vi "运维调试_CODCr.vi"() -> ()   [LabVIEW 2016, in "CODCr库.lvlib"]
uses:
  <vilib>/Utility/miscctls.llb/LVPointTypeDef.ctl
  <vilib>/ptbypt/NI_PtbyPt.lvlib
  <vilib>/Utility/config.llb/NI_LVConfig.lvlib
panel:
  in  "仪器参数":bool
  in  "MB通信方式选择":enum16{"串口", "TCP"}(ring)
  in  "释放串口":bool
  in  "打开串口":bool
  in  "加标回收测试":bool
  in  "平行样测试":bool
  in  "定时启动":bool
  out "COM口":string
  in  "空白测试":bool
  in  "隐藏按钮":bool
  in  "写入消解温度时长":bool
  in  "保存KB值":bool
  in  "标样核查":bool
  out "启动时间":timestamp format="%<%Y/%m/%d %H:%M:%S>T"
  out "主循环次数":i32
  out "status":bool
  out "启动测量模式":T1(ring)
  out "曲线斜率B":sgl format="%#_10g"
  out "曲线斜率K":sgl format="%#_10g"
  out "量程上限":sgl
  out "量程下限":sgl
  out "消解时长":u16
  out "消解温度":u16
  out "测量精度":u16
  out "测量结果":sgl
  out "标样参考值":sgl
  out "量程":u16
  out "工作状态":T1(ring)
  out "仪器时间":timestamp format="%<%X\n%x>T"
  out "关键参数区":T2
  out "状态告警区":T3
  out "测量数据区":T4 {"单位" items=["ug/L", "mg/L", "ppm", "mg/m3", "cm", "ppb", "ug/m3", "%", "nmol/mol", "umol/mol", "MPN/L", "MPN/100ml", "ng/m3", "NTU", "无量纲", "ms/cm", "us/cm", "℃", "mV", "万个/L"]}
  out "系统时间":timestamp format="%<%Y/%m/%d %H:%M:%S>T"
  in  "停止":bool
  in  "校时":bool
  in  "标样校准":bool
  in  "空白校准":bool
  in  "零点核查":bool
  in  "跨度核查":bool
  in  "水样测试":bool
  in  "返回":bool
  in  "设置":bool
  # "mg/L"
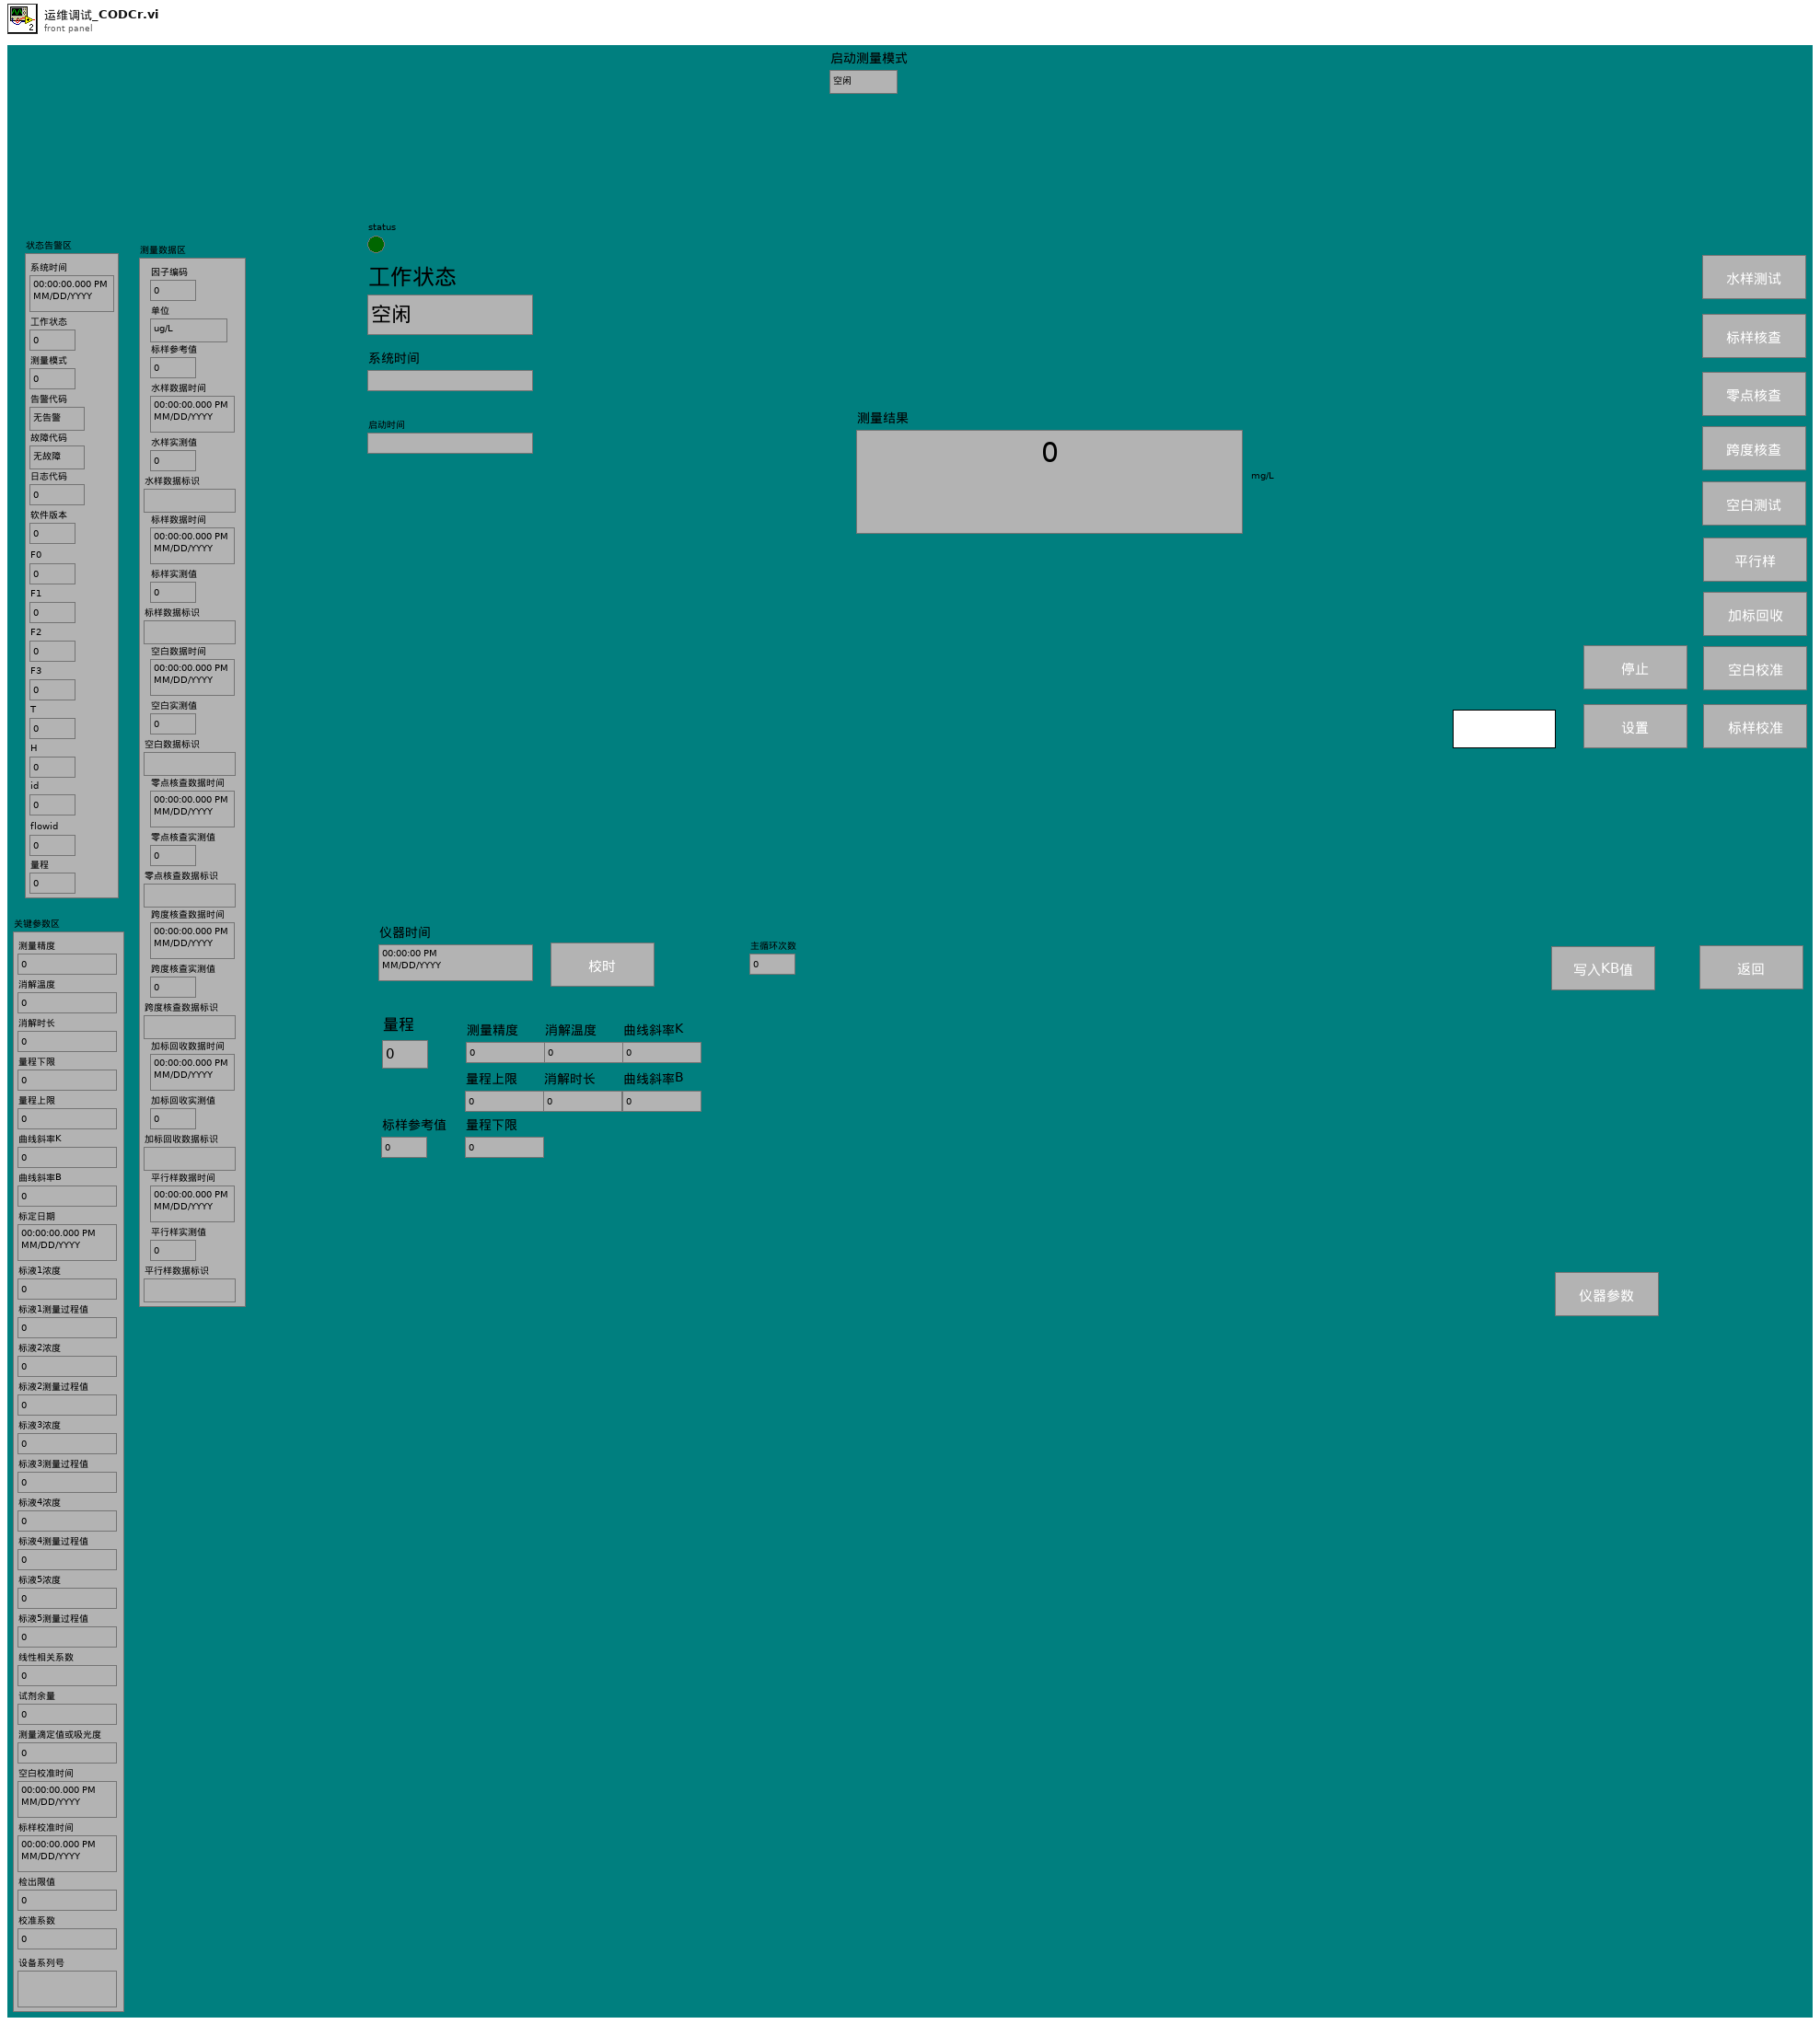
[diagram p1: front panel]
types:
  T1 = enum16{"空闲", "水样测试", "标样核查", "零点核查", "跨度核查", "空白测试", "平行样测试", "加标回收", "空白校准", "标样校准", "初始化（清洗）"}
  T2 = cluster{"测量精度":u16, "消解温度":u16, "消解时长":u16, "量程下限":sgl, "量程上限":sgl, "曲线斜率K":sgl, "曲线斜率B":sgl, "标定日期":timestamp, "标液1浓度":sgl, "标液1测量过程值":sgl, "标液2浓度":sgl, "标液2测量过程值":sgl, "标液3浓度":sgl, "标液3测量过程值":sgl, "标液4浓度":sgl, "标液4测量过程值":sgl, "标液5浓度":sgl, "标液5测量过程值":sgl, "线性相关系数":sgl, "试剂余量":u32, "测量滴定值或吸光度":sgl, "空白校准时间":timestamp, "标样校准时间":timestamp, "检出限值":sgl, "校准系数":sgl, "设备系列号":string}
  T3 = cluster{"系统时间":timestamp, "工作状态":u16, "测量模式":u16, "告警代码":enum16{"无告警", "缺试剂告警", "缺水样告警", "缺蒸馏水告警", "缺标液告警", "仪表漏液告警", "标定异常告警", "超量程告警", "加热异常", "低试剂预警", "超上限告警", "超下限告警", "仪表内部其他异常", "滴定异常告警", "电极异常告警", "量程切换告警", "参数设置告警", "PH电极电位异常", "电导率电极异常", "浊度光度异常", "溶解氧电极异常", "溶解氧光强异常", "温度异常告警", "PH异常告警", "溶解氧异常告警", "电导率异常告警", "浊度异常告警", "叶绿素异常告警", "藻密度异常告警", "蓝绿藻异常告警", "ORP异常告警", "氨氮异常告警", "清洁刷异常告警", "SD卡异常告警", "蓝牙异常告警", "Wifi异常告警", "流程异常告警"}, "故障代码":enum16{"无故障", "电机故障", "温度故障", "通讯故障", "滴定故障"}, "日志代码":u16, "软件版本":u16, "F0":sgl, "F1":sgl, "F2":sgl, "F3":sgl, "T":sgl, "H":sgl, "id":u16, "flowid":u16, "量程":u16}
  T4 = cluster{"因子编码":u32, "单位":u16, "标样参考值":sgl, "水样数据时间":timestamp, "水样实测值":sgl, "水样数据标识":string, "标样数据时间":timestamp, "标样实测值":sgl, "标样数据标识":string, "空白数据时间":timestamp, "空白实测值":sgl, "空白数据标识":string, "零点核查数据时间":timestamp, "零点核查实测值":sgl, "零点核查数据标识":string, "跨度核查数据时间":timestamp, "跨度核查实测值":sgl, "跨度核查数据标识":string, "加标回收数据时间":timestamp, "加标回收实测值":sgl, "加标回收数据标识":string, "平行样数据时间":timestamp, "平行样实测值":sgl, "平行样数据标识":string}
  T5 = cluster{"命令":string, "测量模式":enum16{"水样测量", "标样核查", "零点核查", "跨度核查", "空白测试", "加标回收", "平行样", "校零", "校标"}, "CODCr量程切换":enum32{"H", "L", "AUTO"}}
  T6 = cluster{"测量模式":enum16{"水样测量", "标样核查", "零点核查", "跨度核查", "空白测试", "加标回收", "平行样", "校零", "校标"}}
  T7 = cluster{"仪器测试类型":enum16{"水样测试", "标样核查", "空白测试", "跨度核查"}, "周期设置类型":enum16{"定点启动", "间隔启动"}, "定时功能启用":bool, "定时间隔":dbl, "24H周期设置":bool[]}
  T8 = typedef "LVDateTimeRec.ctl" = cluster{"秒数的小数部分":dbl, "秒":i32, "分":i32, "时":i32, "日":i32, "月":i32, "年":i32, "天数（周）":i32, "天数（年）":i32, "DST":i32}
  T9 = typedef "LVPointTypeDef.ctl" = cluster{"Horizontal":i16, "Vertical":i16}
  T10 = typedef "NI_LVConfig.lvlib/Config Data RefNum.ctl" = refnum<k1>
  T11 = cluster{"运行模式":enum16{"维护模式", "常规模式", "应急模式", "质控模式"}}
  T12 = cluster{"时间标识":timestamp, "监测值":sgl, "单位":u16, "数据标识":string, "因子编码":u32, "标样参考值":sgl, "F0":sgl, "F1":sgl, "F2":sgl, "F3":sgl, "温度":sgl, "湿度":sgl, "量程标识":string}
  T13 = cluster{"时间标识":timestamp, "设备":string, "日志信息":string}
  T14 = cluster{"时间标识":timestamp, "参数":string, "日志信息":string, "流程参数":string}
  T15 = enum16{"无告警", "缺试剂告警", "缺水样告警", "缺蒸馏水告警", "缺标液告警", "仪表漏液告警", "标定异常告警", "超量程告警", "加热异常", "低试剂预警", "超上限告警", "超下限告警", "仪表内部其他异常", "滴定异常告警", "电极异常告警", "量程切换告警", "参数设置告警", "PH电极电位异常", "电导率电极异常", "浊度光度异常", "溶解氧电极异常", "溶解氧光强异常", "温度异常告警", "PH异常告警", "溶解氧异常告警", "电导率异常告警", "浊度异常告警", "叶绿素异常告警", "藻密度异常告警", "蓝绿藻异常告警", "ORP异常告警", "氨氮异常告警", "清洁刷异常告警", "SD卡异常告警", "蓝牙异常告警", "Wifi异常告警", "流程异常告警"}
  T16 = cluster{"时间标识":timestamp, "设备":string, "日志信息":string, "流程参数":string}
  T17 = enum16{"水样测量", "标样核查", "零点核查", "跨度核查", "空白测试", "加标回收", "平行样", "校零", "校标"}
  T18 = cluster{"测量量程":dbl, "测量精度":dbl, "测量间隔":dbl, "消解温度":dbl, "消解时长":dbl, "空白校准时间":timestamp, "曲线截距":dbl, "曲线斜率":dbl, "测量检出限":dbl, "测量信号值":dbl, "线性相关系数":dbl, "二次多项式系数":dbl, "标样校准时间":timestamp, "单位":u16}
  T19 = cluster{"确定":bool, "测量量程":dbl, "测量精度":dbl, "测量间隔":dbl, "消解温度":dbl, "消解时长":dbl, "空白校准时间":timestamp, "曲线截距":dbl, "曲线斜率":dbl, "测量检出限":dbl, "测量信号值":dbl, "线性相关系数":dbl, "二次多项式系数":dbl, "标样校准时间":timestamp, "单位":u16}
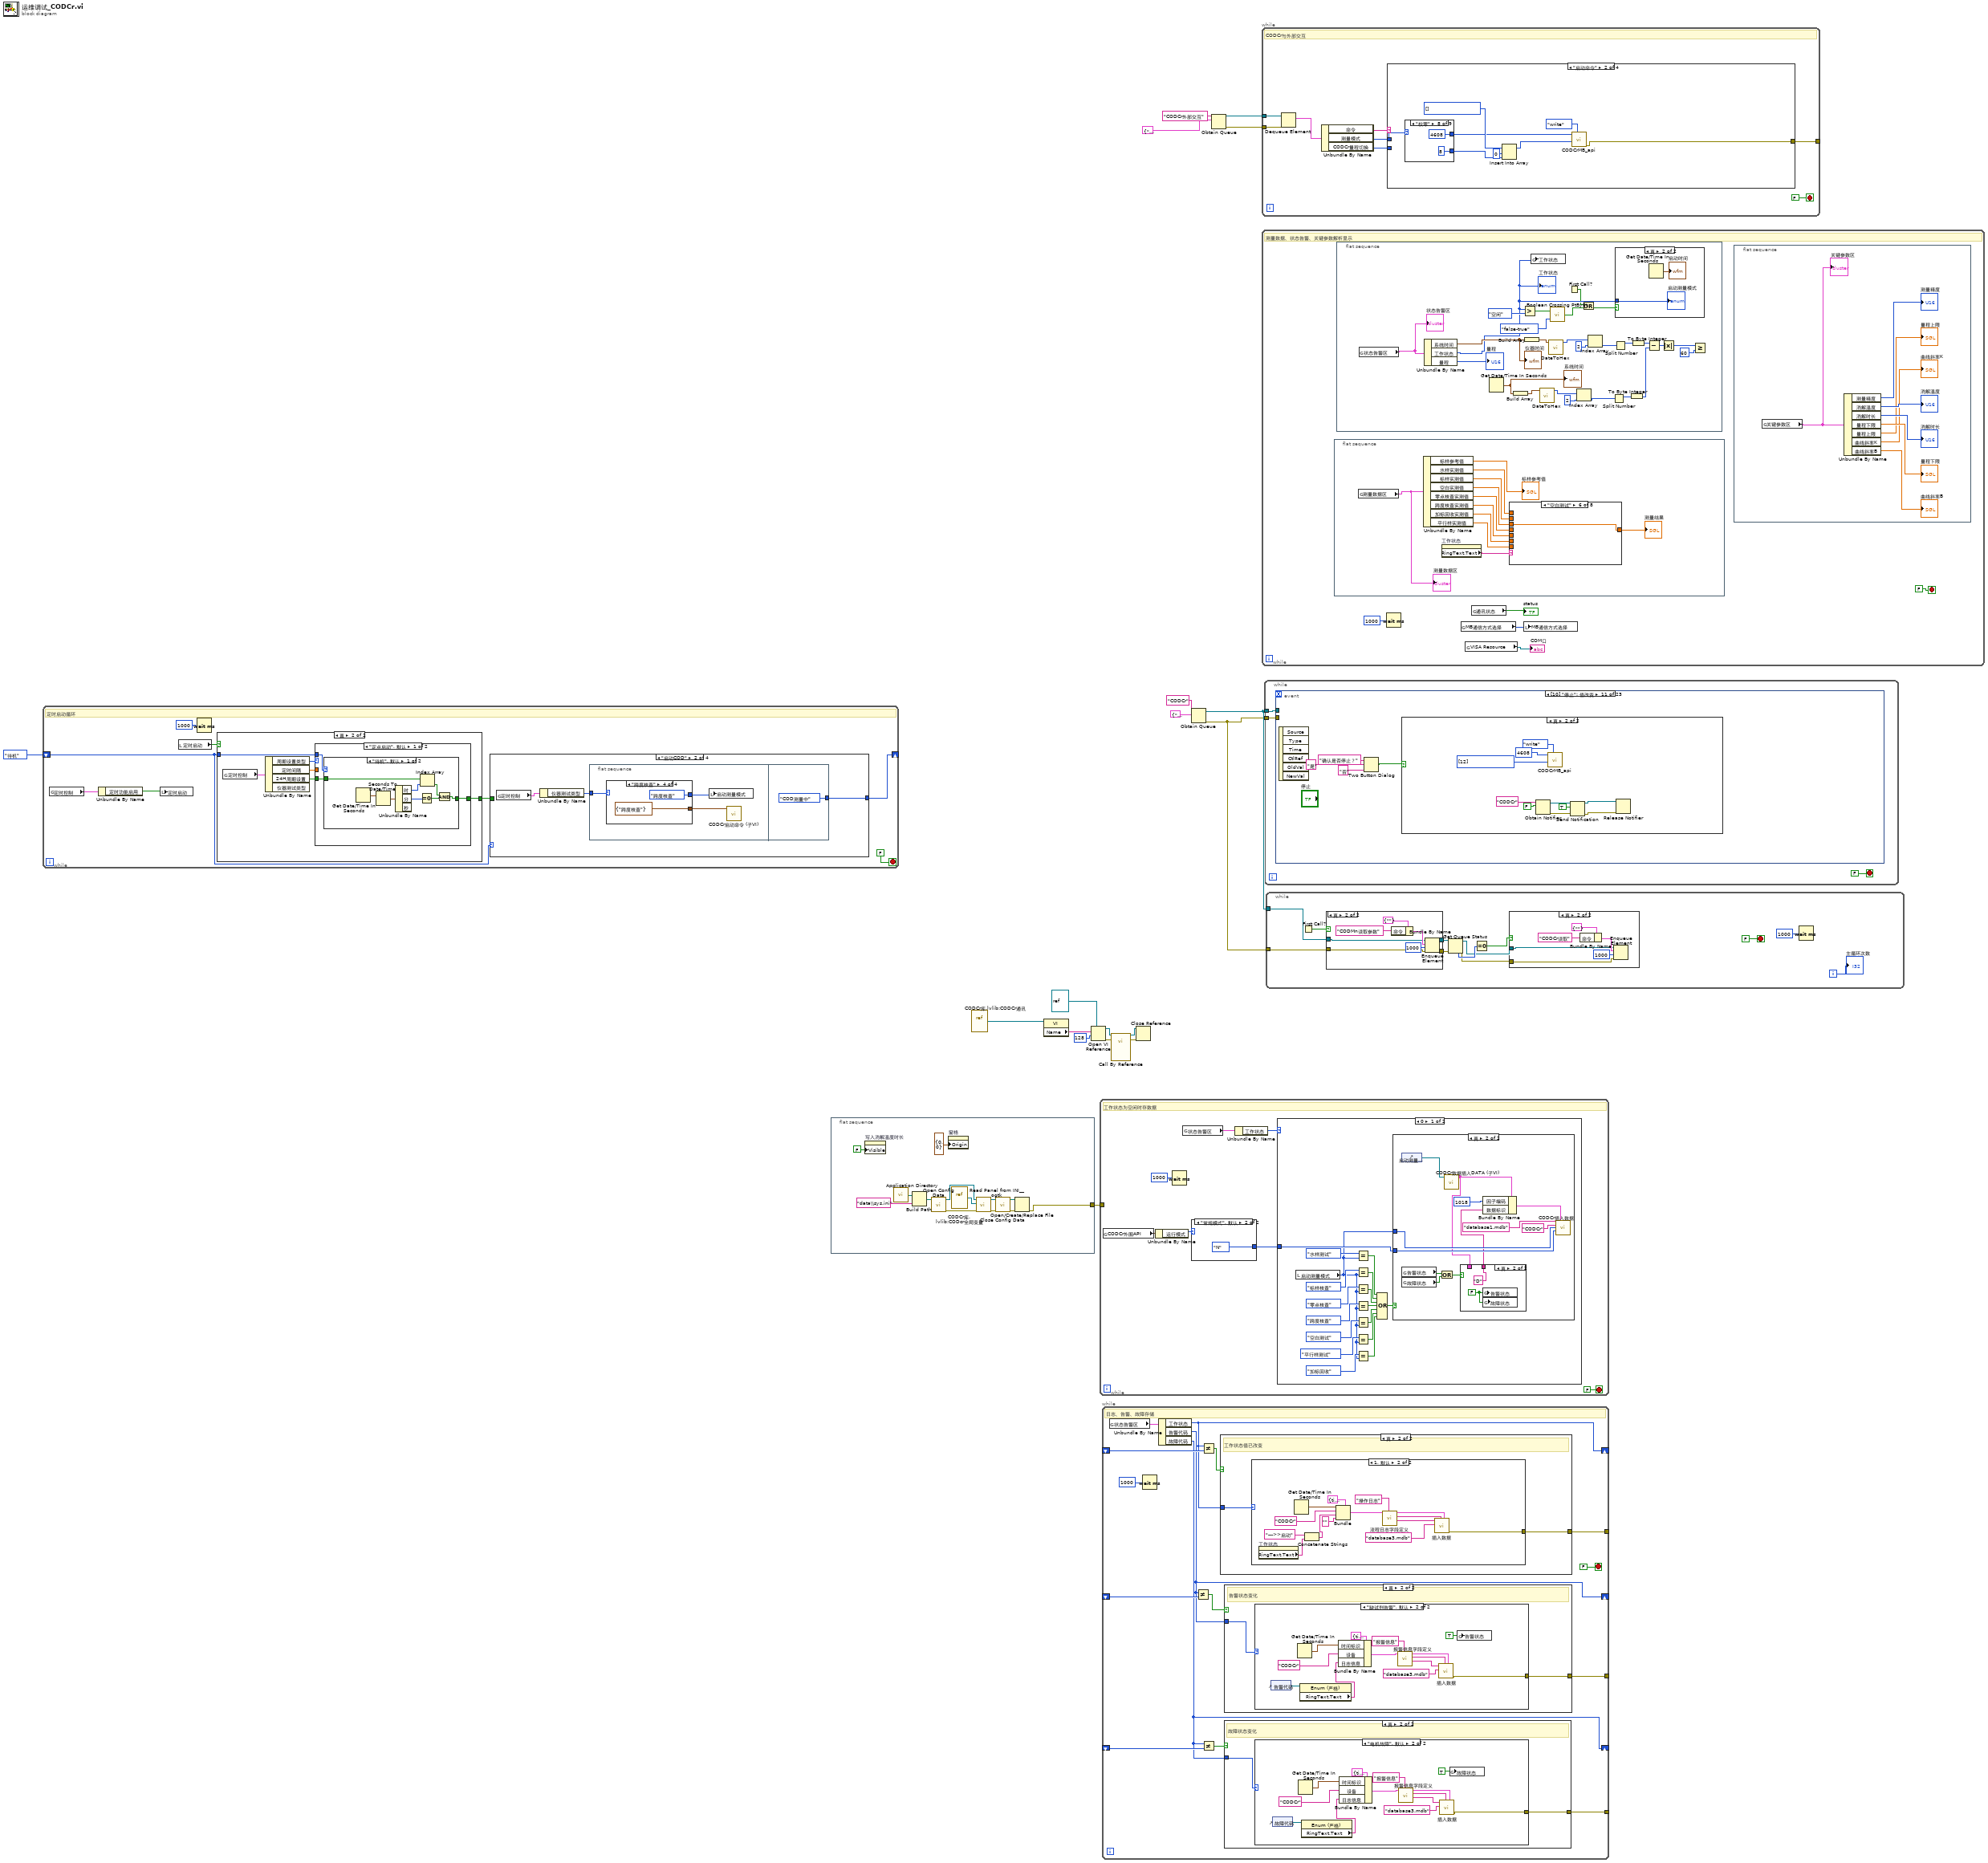
[diagram p0: block diagram]
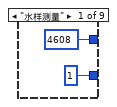
[diagram p5: hidden frame]
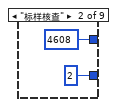
[diagram p6: hidden frame]
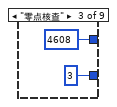
[diagram p7: hidden frame]
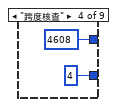
[diagram p8: hidden frame]
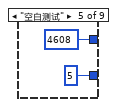
[diagram p9: hidden frame]
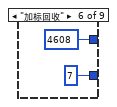
[diagram p10: hidden frame]
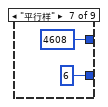
[diagram p11: hidden frame]
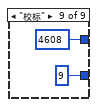
[diagram p12: hidden frame]
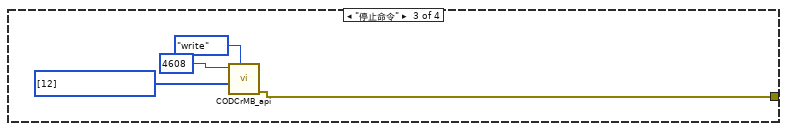
[diagram p13: hidden frame]
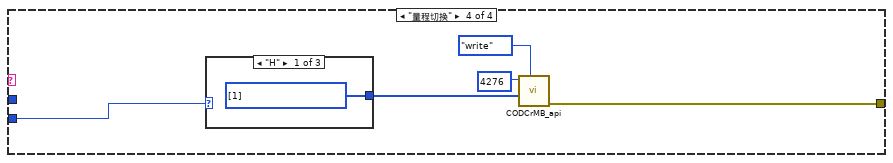
[diagram p14: hidden frame]
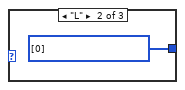
[diagram p15: hidden frame]
diagram:
  n1 = while {
    shift-right: [w24] -> _
    shift-left: enum16{"待机", "启动COD", "COD测量中", "延时"}."待机" -> [w23]
    stop <- FALSE stop-if-true
    # "定时启动循环"
    n2 = global read "CODcr全局变量.vi" "定时控制"() -> (w20:T7)
    n3 = Unbundle By Name(w20) -> ("定时功能启用"=w19:bool)
    n4 = local write "定时启动"(w19) -> ()
    n5 = local read "定时启动"() -> (w21:bool)
    n6 = Wait (ms)(milliseconds to wait=u32 1000 ("等待时间（毫秒）")) -> ()  [unwired: 1 out]
    n7 = case shown="真" w21 {
      tunnel: w23 -> [_ w59]
      tunnel: [_ w58] -> w22
      frame False {
      }
      frame True {
        n8 = global read "CODcr全局变量.vi" "定时控制"() -> (w57:T7)
        n9 = Unbundle By Name(w57) -> ("周期设置类型"=w60:enum16{"定点启动", "间隔启动"}, "定时间隔"=w61:dbl, "24H周期设置"=w62:bool[])  [unwired: 1 out]
        n10 = case shown="\"定点启动\", 默认" w60 {
          tunnel: w61 -> [_ w77]
          tunnel: w62 -> [w65 _]
          tunnel: w59 -> [w63 w80]
          tunnel: [w64 w75] -> w58
          frame "定点启动", Default {
            n11 = case shown="\"待机\", 默认" w63 {
              tunnel: w65 -> [w71 _]
              tunnel: [w66 _] -> w64
              frame "待机", Default {
                n12 = Get Date/Time In Seconds() -> (seconds since 1Jan1904=w73:timestamp)
                n13 = Seconds To Date/Time(time stamp (now)=w73) -> (date time rec=w72:T8)  [unwired: 1 in]
                n14 = Unbundle By Name(w72) -> ("时"=w70:i32, "分"=w69:i32)  [unwired: 1 out]
                n15 = Equal To 0?(x=w69) -> (x = 0?=w67:bool)
                n16 = Index Array(array=w71, index=w70) -> (element=w68:bool)
                n17 = Compound Arithmetic op=AND ("复合运算")(w68, w67) -> (w66:bool)
              }
              frame "启动COD" {
              }
            }
          }
          frame "间隔启动" {
            n18 = Multiply(x=w77, y=60.0) -> (x*y=w74:dbl)
            n19 = feedback #1(w74) -> (w79:dbl)
            n20 = case shown="\"待机\"" w80 {
              tunnel: w79 -> [_ w82]
              tunnel: [_ w81] -> w78
              frame Default {
              }
              frame "待机" {
                n21 = Increment(x=w82) -> (x+1=w81:dbl)
              }
            }
            n22 = feedback-in #1(w78) -> ()
            n23 = Greater Or Equal?(x=w78, y=w74) -> (x >= y?=w75:bool)
          }
        }
      }
    }
    n24 = case shown="\"启动COD\"" w23 {
      tunnel: [w27 w33 w47 enum16{"待机", "启动COD", "COD测量中", "延时"}."待机"] -> w24
      tunnel: w22 -> [w30 _ _ _]
      frame "待机", Default {
        n25 = Select(t=enum16{"待机", "启动COD", "COD测量中", "延时"}."启动COD", s=w30, f=enum16{"待机", "启动COD", "COD测量中", "延时"}."待机") -> (s? t:f=w27:enum16{"待机", "启动COD", "COD测量中", "延时"})
      }
      frame "启动COD" {
        n26 = global read "CODcr全局变量.vi" "定时控制"() -> (w31:T7)
        n27 = Unbundle By Name(w31) -> ("仪器测试类型"=w32:enum16{"水样测试", "标样核查", "空白测试", "跨度核查"})
        n28 = flat-sequence {
          tunnel: w32 -> [w36]
          tunnel: [enum16{"待机", "启动COD", "COD测量中", "延时"}."COD测量中"] -> w33
          frame #0 {
            n29 = case shown="\"跨度核查\"" w36 {
              tunnel: [T6 {"测量模式"=enum."水样测量"} ("启动测量模式") T6 {"测量模式"=enum."标样核查"} ("启动测量模式") T6 {"测量模式"=enum."空白测试"} ("启动测量模式") T6 {"测量模式"=enum."跨度核查"} ("启动测量模式")] -> w35
              tunnel: [T1."水样测试" ("启动测量模式") T1."标样核查" ("启动测量模式") T1."空白测试" ("启动测量模式") T1."跨度核查" ("启动测量模式")] -> w34
              frame "水样测试", Default {
              }
              frame "标样核查" {
              }
              frame "空白测试" {
              }
              frame "跨度核查" {
              }
            }
            n30 = local write "启动测量模式"(w34) -> ()
            n31 = call "CODCr启动命令 (子VI).vi"("启动测量模式"=w35) -> ()  [unwired: 11 in]
          }
          frame #1 {
          }
        }
      }
      frame "COD测量中" {
        n32 = flat-sequence {
          tunnel: [w51] -> w46
          tunnel: [w55] -> w47
          tunnel: w46 -> [w55]
          frame #0 {
            n33 = local read "状态告警区"() -> (w50:T3)
            n34 = Unbundle By Name(w50) -> ("工作状态"=w49:u16)
            n35 = Equal To 0?(x=w49) -> (x = 0?=w48:bool)
            n36 = Select(t=enum16{"待机", "启动COD", "COD测量中", "延时"}."延时", s=w48, f=enum16{"待机", "启动COD", "COD测量中", "延时"}."COD测量中") -> (s? t:f=w51:enum16{"待机", "启动COD", "COD测量中", "延时"})
          }
          frame #1 {
            n37 = Wait (ms)(milliseconds to wait=u32 5000 ("等待时间（毫秒）")) -> ()  [unwired: 1 out]
          }
        }
      }
      frame "延时" {
      }
    }
  }
  n38 = flat-sequence {
    tunnel: [w83] -> w17
    frame #0 {
      n39 = property on="写入消解温度时长" class="Bool"("Visible"=FALSE ("可见")) -> ()  [unwired: 2 in, 2 out]
      n40 = call <vilib>:"Application Directory.vi"() -> ("Application Directory"=w93:path)
      n41 = Build Path(base path=w93, name or relative path="data\\sys.ini" ("名称或相对路径")) -> (appended path=w91:path)
      n42 = call <vilib>:"Open Config Data.vi"("configuration file path"=w91) -> ("error out"=w87:errorcluster, "refnum"=w90:T10)  [unwired: 8 in, 1 out]
      n43 = property on="窗格" class="Pane"("Origin"=T9 {"Horizontal"=0, "Vertical"=0} ("原点")) -> ()  [unwired: 2 in, 2 out]
      n44 = vi-ref "CODCr库.lvlib:CODcr全局变量.vi"() -> (w89:refnum<vi>)
      n45 = call <userlib>:"Read Panel from INI__ogtk.vi"("error in (no error)"=w87, "VI ref"=w89, "refnum"=w90) -> ("error out"=w86:errorcluster, "refnum out"=w88:T10)  [unwired: 7 in]
      n46 = call <vilib>:"Close Config Data.vi"("error in (no error)"=w86, "refnum"=w88) -> ("error out"=w85:errorcluster, "file path"=w84:path)  [unwired: 8 in]
      n47 = Open/Create/Replace File(file path (use dialog)=w84, error in=w85) -> (error out=w83:errorcluster)  [unwired: 4 in, 2 out]
    }
  }
  n48 = vi-ref "CODCr库.lvlib:CODCr通讯.vi"() -> (w9:refnum<vi>)
  n49 = property class="VI"(reference=w9) -> ("Name"=w10:string)  [unwired: 1 in, 2 out]
  n50 = Open VI Reference(type specifier VI Refnum (for type only)=refnum<vi> refnum, vi path=w10, options=128 ("选项")) -> (vi reference=w12:refnum<vi>, error out=w14:errorcluster)  [unwired: 3 in]
  n51 = while "While循环" {
    tunnel: w17 -> [_]
    stop <- FALSE stop-if-true
    # "工作状态为空闲时存数据"
    n52 = global read "CODCr外部API.vi" "CODCr外围API"() -> (w98:T11)
    n53 = Unbundle By Name(w98) -> ("运行模式"=w97:enum16{"维护模式", "常规模式", "应急模式", "质控模式"})
    n54 = Wait (ms)(milliseconds to wait=u32 1000 ("等待时间（毫秒）")) -> ()  [unwired: 1 out]
    n55 = global read "CODcr全局变量.vi" "状态告警区"() -> (w96:T3)
    n56 = case shown="\"常规模式\", 默认" w97 {
      tunnel: [enum16{"N", "M"}."M" ("数据类型") enum16{"N", "M"}."N" ("数据类型")] -> w99
      frame "维护模式" {
      }
      frame "常规模式", Default {
      }
    }
    n57 = Unbundle By Name(w96) -> ("工作状态"=w100:u16)
    n58 = case shown="0" w100 {
      tunnel: w99 -> [w121 _]
      frame 0 {
        n59 = local read "启动测量模式"() -> (w113:T1)
        n60 = Equal?(x=T1."水样测试" ("启动测量模式"), y=w113) -> (x = y?=w112:bool)
        n61 = Equal?(x=T1."标样核查" ("启动测量模式"), y=w113) -> (x = y?=w111:bool)
        n62 = Equal?(x=T1."零点核查" ("启动测量模式"), y=w113) -> (x = y?=w110:bool)
        n63 = Equal?(x=T1."跨度核查" ("启动测量模式"), y=w113) -> (x = y?=w109:bool)
        n64 = Equal?(x=T1."空白测试" ("启动测量模式"), y=w113) -> (x = y?=w108:bool)
        n65 = Equal?(x=T1."平行样测试" ("启动测量模式"), y=w113) -> (x = y?=w107:bool)
        n66 = Equal?(x=T1."加标回收" ("启动测量模式"), y=w113) -> (x = y?=w106:bool)
        n67 = Compound Arithmetic op=OR(w112, w111, w110, w109, w108, w107, w106) -> (w105:bool)
        n68 = case shown="真" w105 {
          tunnel: w113 -> [_ w129]
          tunnel: w121 -> [_ w128]
          frame False {
          }
          frame True {
            n69 = control-ref of="启动测量模式"() -> (w133:refnum<vi>)
            n70 = global read "CODcr全局变量.vi" "告警状态"() -> (w126:bool)
            n71 = global read "CODcr全局变量.vi" "故障状态"() -> (w125:bool)
            n72 = Or(x=w126, y=w125) -> (x .or. y?=w124:bool)
            n73 = call "CODCr数据插入DATA (子VI).vi"("Enum输入"=w133) -> ("data"=w123:T12)  [unwired: 10 in]
            n74 = case shown="真" w124 {
              tunnel: w123 -> [w135 _]
              tunnel: [w134 "D" ("table")] -> w122
              frame False {
                n75 = Unbundle By Name(w135) -> ("数据标识"=w134:string)
              }
              frame True {
                w136 = FALSE ("告警状态")
                n76 = global write "CODcr全局变量.vi" "告警状态"(w136) -> ()
                n77 = global write "CODcr全局变量.vi" "故障状态"(w136) -> ()
              }
            }
            n78 = Bundle By Name(cluster=w123, "因子编码"=u32 1018, "数据标识"=w122) -> (w132:T12)
            n79 = call "CODCr插入数据.vi"("database"="database1.mdb", "data"=w132, "table"="CODCr", "测量模式"=w129, "数据类型"=w128) -> ()  [unwired: 10 in, 1 out]
          }
        }
      }
      frame 1, Default {
      }
    }
  }
  n80 = while {
    shift-right: [w148] -> _
    shift-left: _ -> [w150]
    tunnel: [w147] -> _
    shift-right: [w143] -> _
    shift-left: _ -> [w144]
    shift-right: [w139] -> _
    shift-left: _ -> [w141]
    tunnel: [w140] -> _
    tunnel: [w138] -> _
    stop <- FALSE stop-if-true
    # "日志、告警、故障存储"
    n81 = global read "CODcr全局变量.vi" "状态告警区"() -> (w146:T3)
    n82 = Wait (ms)(milliseconds to wait=u32 1000 ("等待时间（毫秒）")) -> ()  [unwired: 1 out]
    n83 = Unbundle By Name(w146) -> ("工作状态"=w148:u16, "告警代码"=w143:T15, "故障代码"=w139:enum16{"无故障", "电机故障", "温度故障", "通讯故障", "滴定故障"})
    n84 = Not Equal?(x=w143, y=w144) -> (x != y?=w145:bool)
    n85 = Not Equal?(x=w148, y=w150) -> (x != y?=w149:bool)
    n86 = Not Equal?(x=w139, y=w141) -> (x != y?=w142:bool)
    n87 = case shown="真" w149 {
      tunnel: w148 -> [_ w184]
      tunnel: [_ w183] -> w147
      frame False {
      }
      frame True {
        # "工作状态值已改变"
        n88 = case shown="1, 默认" w184 {
          tunnel: [w185 w200] -> w183
          frame 0 {
            n89 = Get Date/Time In Seconds() -> (seconds since 1Jan1904=w192:timestamp)
            n90 = Bundle(cluster=T14 {"时间标识"=timestamp(0 s since 1904-01-01), "参数"="", "日志信息"="", "流程参数"=""} ("data in"), "时间标识"=w192, "参数"="CODCr" ("table输入"), "日志信息"="--->>结束", "流程参数"="" ("table输入")) -> (w186:T14)
            n91 = call "流程日志字段定义.vi"("table输入"="操作日志", "data in"=w186) -> ("table输出"=w190:string, "columns"=w188:string[], "data out"=w187:T16)  [unwired: 7 in]
            n92 = call "插入数据.vi"("data"=w187, "columns"=w188, "database"="database3.mdb", "table"=w190) -> ("error out"=w185:errorcluster)  [unwired: 7 in]
          }
          frame 1, Default {
            n93 = property on="工作状态" class="Enum (严格)"() -> ("RingText.Text"=w197:string)  [unwired: 2 in, 2 out]
            n94 = Get Date/Time In Seconds() -> (seconds since 1Jan1904=w207:timestamp)
            n95 = Concatenate Strings("--->>启动" ("日志信息"), w197) -> (w198:string)
            n96 = Bundle(cluster=T14 {"时间标识"=timestamp(0 s since 1904-01-01), "参数"="", "日志信息"="", "流程参数"=""} ("data in"), "时间标识"=w207, "参数"="CODCr" ("table输入"), "日志信息"=w198, "流程参数"="" ("table输入")) -> (w206:T14)
            n97 = call "流程日志字段定义.vi"("table输入"="操作日志", "data in"=w206) -> ("table输出"=w204:string, "columns"=w202:string[], "data out"=w201:T16)  [unwired: 7 in]
            n98 = call "插入数据.vi"("data"=w201, "columns"=w202, "database"="database3.mdb", "table"=w204) -> ("error out"=w200:errorcluster)  [unwired: 7 in]
          }
        }
      }
    }
    n99 = case shown="真" w142 {
      tunnel: w139 -> [_ w154]
      tunnel: [_ w153] -> w138
      frame False {
      }
      frame True {
        # "故障状态变化"
        n100 = case shown="\"电机故障\", 默认" w154 {
          tunnel: [_ w156] -> w153
          frame "无故障" {
            # "无告警"
          }
          frame "电机故障", Default {
            n101 = control-ref of="故障代码"() -> (w166:refnum<vi>)
            n102 = Get Date/Time In Seconds() -> (seconds since 1Jan1904=w164:timestamp)
            n103 = property class="Enum (严格)"(reference=w166) -> ("RingText.Text"=w167:string)  [unwired: 1 in, 2 out]
            n104 = Bundle By Name(cluster=T13 {"时间标识"=timestamp(0 s since 1904-01-01), "设备"="", "日志信息"=""} ("data in"), "时间标识"=w164, "设备"="CODCr" ("table输入"), "日志信息"=w167) -> (w163:T13)
            n105 = call "报警信息字段定义.vi"("table输入"="报警信息", "data in"=w163) -> ("table输出"=w158:string, "columns"=w157:string[], "data out"=w160:T13)  [unwired: 7 in]
            n106 = call "插入数据.vi"("data"=w160, "columns"=w157, "database"="database3.mdb", "table"=w158) -> ("error out"=w156:errorcluster)  [unwired: 7 in]
            n107 = global write "CODcr全局变量.vi" "故障状态"(TRUE ("告警状态")) -> ()
          }
        }
      }
    }
    n108 = case shown="真" w145 {
      tunnel: w143 -> [_ w169]
      tunnel: [_ w168] -> w140
      frame False {
      }
      frame True {
        # "告警状态变化"
        n109 = case shown="\"缺试剂告警\", 默认" w169 {
          tunnel: [_ w175] -> w168
          frame "无告警" {
            # "无告警"
          }
          frame "缺试剂告警", Default {
            n110 = control-ref of="告警代码"() -> (w172:refnum<vi>)
            n111 = Get Date/Time In Seconds() -> (seconds since 1Jan1904=w174:timestamp)
            n112 = property class="Enum (严格)"(reference=w172) -> ("RingText.Text"=w171:string)  [unwired: 1 in, 2 out]
            n113 = Bundle By Name(cluster=T13 {"时间标识"=timestamp(0 s since 1904-01-01), "设备"="", "日志信息"=""} ("data in"), "时间标识"=w174, "设备"="CODCr" ("table输入"), "日志信息"=w171) -> (w176:T13)
            n114 = call "报警信息字段定义.vi"("table输入"="报警信息", "data in"=w176) -> ("table输出"=w181:string, "columns"=w182:string[], "data out"=w179:T13)  [unwired: 7 in]
            n115 = call "插入数据.vi"("data"=w179, "columns"=w182, "database"="database3.mdb", "table"=w181) -> ("error out"=w175:errorcluster)  [unwired: 7 in]
            n116 = global write "CODcr全局变量.vi" "告警状态"(TRUE ("告警状态")) -> ()
          }
        }
      }
    }
  }
  n117 = call-by-ref "?"(reference=w12, error in=w14) -> (reference out=w16:refnum<vi>, error out=w15:errorcluster)  [unwired: 12 in]
  n118 = Close Reference(reference=w16, error in (no error)=w15) -> ()  [unwired: 1 out]
  n119 = Obtain Queue(name (unnamed)="CODCr" ("名称（未命名）"), element data type=cluster{"命令":string} {"命令"="启用模块"} ("元素")) -> (queue out=w2:refnum<queue>, error out=w1:errorcluster)  [unwired: 3 in, 1 out]
  n120 = Obtain Queue(name (unnamed)="CODCr外部交互" ("名称（未命名）"), element data type=T5 {"命令"="启动命令", "测量模式"=enum."水样测量", "CODCr量程切换"=enum."AUTO"} ("元素")) -> (queue out=w4:refnum<queue>, error out=w3:errorcluster)  [unwired: 3 in, 1 out]
  n121 = while {
    tunnel: w4 -> [w216]
    tunnel: w3 -> [w215]
    tunnel: [w211] -> _
    stop <- FALSE stop-if-true
    # "CODCr与外部交互"
    n122 = Dequeue Element(queue=w216, error in (no error)=w215) -> (element=w217:T5)  [unwired: 1 in, 3 out]
    n123 = Unbundle By Name(w217) -> ("命令"=w214:string, "测量模式"=w213:T17, "CODCr量程切换"=w212:enum32{"H", "L", "AUTO"})
    n124 = case shown="\"启动命令\"" w214 {
      tunnel: w213 -> [_ w220 _ _]
      tunnel: w212 -> [_ _ _ w250]
      tunnel: [_ w219 w245 w249] -> w211
      frame "假", Default {
      }
      frame "启动命令" {
        n125 = case shown="\"校零\"" w220 {
          tunnel: [u16 4608 ("address") u16 4608 ("address") u16 4608 ("address") u16 4608 ("address") u16 4608 ("address") u16 4608 ("address") u16 4608 ("address") u16 4608 ("address") u16 4608 ("address")] -> w222
          tunnel: [u16 1 ("address") u16 2 ("address") u16 3 ("address") u16 4 ("address") u16 5 ("address") u16 7 ("address") u16 6 ("address") u16 8 ("address") u16 9 ("address")] -> w226
          frame "水样测量" {
          }
          frame "标样核查" {
          }
          frame "零点核查" {
          }
          frame "跨度核查" {
          }
          frame "空白测试" {
          }
          frame "加标回收" {
          }
          frame "平行样" {
          }
          frame "校零" {
          }
          frame "校标" {
          }
        }
        n126 = Insert Into Array(array=u16[] [] ("values"), index=0 ("索引"), new element=w226) -> (w221:u16[])
        n127 = call "CODCrMB_api.vi"("STEP"=enum16{"open", "read", "write", "close"}."write", "values"=w221, "starting address"=w222) -> ("error out"=w219:errorcluster)  [unwired: 6 in, 2 out]
      }
      frame "停止命令" {
        n128 = call "CODCrMB_api.vi"("STEP"=enum16{"open", "read", "write", "close"}."write", "values"=u16[] [12], "starting address"=u16 4608) -> ("error out"=w245:errorcluster)  [unwired: 6 in, 2 out]
      }
      frame "量程切换" {
        n129 = case shown="\"H\"" w250 {
          tunnel: [u16[] [1] ("values") u16[] [0] ("values") _] -> w253
          frame "H" {
          }
          frame "L" {
          }
          frame "AUTO", Default {
          }
        }
        n130 = call "CODCrMB_api.vi"("STEP"=enum16{"open", "read", "write", "close"}."write", "values"=w253, "starting address"=u16 4276) -> ("error out"=w249:errorcluster)  [unwired: 6 in, 2 out]
      }
    }
  }
  n131 = while {
    stop <- FALSE stop-if-true
    # "测量数据、状态告警、关键参数解析显示"
    n132 = flat-sequence {
      frame #0 {
        n133 = global read "CODcr全局变量.vi" "测量数据区"() -> (w297:T4)
        "测量数据区" <- w297
        n134 = Unbundle By Name(w297) -> ("标样参考值"=→"标样参考值":sgl, "水样实测值"=w305:sgl, "标样实测值"=w303:sgl, "空白实测值"=w300:sgl, "零点核查实测值"=w302:sgl, "跨度核查实测值"=w301:sgl, "加标回收实测值"=w298:sgl, "平行样实测值"=w299:sgl)
        n135 = property on="工作状态" class="Enum (严格)"() -> ("RingText.Text"=w306:string)  [unwired: 2 in, 2 out]
        n136 = case shown="\"空白测试\"" w306 {
          tunnel: w305 -> [_ w309 _ _ _ _ _ _]
          tunnel: [w308 w309 w310 w311 w312 w313 w314 w315] -> w304
          tunnel: w303 -> [_ _ w310 _ _ _ _ _]
          tunnel: w302 -> [_ _ _ w311 _ _ _ _]
          tunnel: w301 -> [_ _ _ _ w312 _ _ _]
          tunnel: w300 -> [_ _ _ _ _ w313 _ _]
          tunnel: w299 -> [_ _ _ _ _ _ w314 _]
          tunnel: w298 -> [_ _ _ _ _ _ _ w315]
          frame "空闲", Default {
            n137 = local read "测量结果"() -> (w308:sgl)
          }
          frame "水样测试" {
          }
          frame "标样核查" {
          }
          frame "零点核查" {
          }
          frame "跨度核查" {
          }
          frame "空白测试" {
          }
          frame "平行样测试" {
          }
          frame "加标回收" {
          }
        }
        "测量结果" <- w304
      }
    }
    n138 = flat-sequence {
      frame #0 {
        n139 = global read "CODcr全局变量.vi" "状态告警区"() -> (w269:T3)
        "状态告警区" <- w269
        n140 = Unbundle By Name(w269) -> ("系统时间"=w281:timestamp, "工作状态"=w272:u16, "量程"=→"量程":u16)
        "仪器时间" <- w281
        "工作状态" <- w272
        n141 = Get Date/Time In Seconds() -> (seconds since 1Jan1904=w282:timestamp)
        "系统时间" <- w282
        n142 = Build Array(w282) -> (w276:timestamp[])
        n143 = Greater?(x=w272, y=T1."空闲") -> (0:w280:bool)
        n144 = Build Array(w281) -> (w275:timestamp[])
        n145 = global write "CODcr全局变量.vi" "工作状态"(w272) -> ()
        n146 = call "DateToHex.vi"("DATE"=w276) -> ("数组"=w273:u16[])  [unwired: 10 in]
        n147 = call "DateToHex.vi"("DATE"=w275) -> ("数组"=w274:u16[])  [unwired: 10 in]
        n148 = call <vilib>:"Boolean Crossing PtByPt.vi"("direction"=enum16{"either", "false-true", "true-false"}."false-true", "input"=w280) -> ("crossing"=w279:bool)  [unwired: 1 in]
        n149 = First Call?() -> (First Call?: T/F=w270:bool)
        n150 = Index Array(array=w273, index=2 ("索引")) -> (element=w284:u16)
        n151 = Or(x=w270, y=w279) -> (x .or. y?=w271:bool)
        n152 = Index Array(array=w274, index=2 ("索引")) -> (element=w285:u16)
        n153 = Split Number(x=w284) -> (hi(x)=w287:u8)  [unwired: 1 out]
        n154 = Split Number(x=w285) -> (hi(x)=w290:u8)  [unwired: 1 out]
        n155 = case shown="真" w271 {
          tunnel: w272 -> [_ w295]
          frame False {
          }
          frame True {
            n156 = Get Date/Time In Seconds() -> (seconds since 1Jan1904=→"启动时间":timestamp)
            "启动测量模式" <- w295
          }
        }
        n157 = To Byte Integer(number=w287) -> (8bit integer=w288:i8)
        n158 = To Byte Integer(number=w290) -> (8bit integer=w291:i8)
        n159 = Subtract(x=w291, y=w288) -> (x-y=w289:i8)
        n160 = Absolute Value(x=w289) -> (abs(x)=w292:i8)
        n161 = Greater Or Equal?(x=w292, y=i8 60) -> ()  [unwired: 1 out]
      }
    }
    n162 = Wait (ms)(milliseconds to wait=u32 1000 ("等待时间（毫秒）")) -> ()  [unwired: 1 out]
    n163 = global read "CODcr全局变量.vi" "MB通信方式选择"() -> (w257:enum16{"串口", "TCP"})
    n164 = global read "CODcr全局变量.vi" "VISA Resource"() -> (→"COM口":refnum<visa-resource-name>)
    n165 = global read "CODcr全局变量.vi" "通讯状态"() -> (→"status":bool)
    n166 = local write "MB通信方式选择"(w257) -> ()
    n167 = flat-sequence {
      frame #0 {
        n168 = global read "CODcr全局变量.vi" "关键参数区"() -> (w261:T2)
        "关键参数区" <- w261
        n169 = Unbundle By Name(w261) -> ("测量精度"=→"测量精度":u16, "消解温度"=→"消解温度":u16, "消解时长"=→"消解时长":u16, "量程下限"=→"量程下限":sgl, "量程上限"=→"量程上限":sgl, "曲线斜率K"=→"曲线斜率K":sgl, "曲线斜率B"=→"曲线斜率B":sgl)
      }
    }
  }
  n170 = while {
    tunnel: w2 -> [w317]
    tunnel: w1 -> [w316]
    stop <- FALSE stop-if-true
    n171 = event shown="[10] \"停止\": 值改变" {
      selector: _ -> [_ _ _ _ _ _ _ _ _ _ _ _ _ _ _ _ _ _ _ _ _ _ _]
      dyn-events: _ -> [_ _ _ _ _ _ _ _ _ _ _ _ _ _ _ _ _ _ _ _ _ _ _]
      timeout: _ -> [_ _ _ _ _ _ _ _ _ _ _ _ _ _ _ _ _ _ _ _ _ _ _]
      tunnel: w317 -> [_ _ _ _ _ _ _ _ _ _ _ _ _ _ w428 w445 _ _ _ w483 _ _ _]
      tunnel: w316 -> [_ _ _ _ _ _ _ _ _ _ _ _ _ _ w427 w444 _ _ _ w482 _ _ _]
      event Timeout {
        n172 = event-data() -> ()  [unwired: 1 in, 2 out]
      }
      event "水样测试": Value Change {
        n173 = event-data() -> ()  [unwired: 1 in, 6 out]
        n174 = local write "启动测量模式"(T1."水样测试" ("启动测量模式")) -> ()
        n175 = call "CODCrMB_api.vi"("STEP"=enum16{"open", "read", "write", "close"}."write", "values"=u16[] [1], "starting address"=u16 4608) -> ()  [unwired: 6 in, 3 out]
      }
      event "标样核查": Value Change {
        n176 = event-data() -> ()  [unwired: 1 in, 6 out]
        n177 = local write "启动测量模式"(T1."标样核查" ("启动测量模式")) -> ()
        n178 = call "CODCrMB_api.vi"("STEP"=enum16{"open", "read", "write", "close"}."write", "values"=u16[] [2], "starting address"=u16 4608) -> ()  [unwired: 6 in, 3 out]
      }
      event "零点核查": Value Change {
        n179 = event-data() -> ()  [unwired: 1 in, 6 out]
        n180 = local write "启动测量模式"(T1."零点核查" ("启动测量模式")) -> ()
        n181 = call "CODCrMB_api.vi"("STEP"=enum16{"open", "read", "write", "close"}."write", "values"=u16[] [3], "starting address"=u16 4608) -> ()  [unwired: 6 in, 3 out]
      }
      event "跨度核查": Value Change {
        n182 = event-data() -> ()  [unwired: 1 in, 6 out]
        n183 = local write "启动测量模式"(T1."跨度核查" ("启动测量模式")) -> ()
        n184 = call "CODCrMB_api.vi"("STEP"=enum16{"open", "read", "write", "close"}."write", "values"=u16[] [4], "starting address"=u16 4608) -> ()  [unwired: 6 in, 3 out]
      }
      event "空白测试": Value Change {
        n185 = event-data() -> ()  [unwired: 1 in, 6 out]
        n186 = local write "启动测量模式"(T1."空白测试" ("启动测量模式")) -> ()
        n187 = call "CODCrMB_api.vi"("STEP"=enum16{"open", "read", "write", "close"}."write", "values"=u16[] [5], "starting address"=u16 4608) -> ()  [unwired: 6 in, 3 out]
      }
      event "平行样测试": Value Change {
        n188 = event-data() -> ()  [unwired: 1 in, 6 out]
        n189 = local write "启动测量模式"(T1."平行样测试" ("启动测量模式")) -> ()
        n190 = call "CODCrMB_api.vi"("STEP"=enum16{"open", "read", "write", "close"}."write", "values"=u16[] [6], "starting address"=u16 4608) -> ()  [unwired: 6 in, 3 out]
      }
      event "加标回收测试": Value Change {
        n191 = event-data() -> ()  [unwired: 1 in, 6 out]
        n192 = local write "启动测量模式"(T1."加标回收" ("启动测量模式")) -> ()
        n193 = call "CODCrMB_api.vi"("STEP"=enum16{"open", "read", "write", "close"}."write", "values"=u16[] [7], "starting address"=u16 4608) -> ()  [unwired: 6 in, 3 out]
      }
      event "空白校准": Value Change {
        n194 = event-data() -> ()  [unwired: 1 in, 6 out]
        n195 = local write "启动测量模式"(T1."空白校准" ("启动测量模式")) -> ()
        n196 = call "CODCrMB_api.vi"("STEP"=enum16{"open", "read", "write", "close"}."write", "values"=u16[] [8], "starting address"=u16 4608) -> ()  [unwired: 6 in, 3 out]
      }
      event "标样校准": Value Change {
        n197 = event-data() -> ()  [unwired: 1 in, 6 out]
        n198 = local write "启动测量模式"(T1."标样校准" ("启动测量模式")) -> ()
        n199 = call "CODCrMB_api.vi"("STEP"=enum16{"open", "read", "write", "close"}."write", "values"=u16[] [9], "starting address"=u16 4608) -> ()  [unwired: 6 in, 3 out]
      }
      event "停止": Value Change {
        n200 = event-data() -> ()  [unwired: 1 in, 6 out]
        n201 = Two Button Dialog(message="确认是否停止？" ("消息"), 1:"否" ("F按钮名称（“取消”）"), 2:"是" ("T按钮名称（“确定”）")) -> (T button?=w355:bool)
        n202 = case shown="真" w355 {
          frame False {
          }
          frame True {
            n203 = Obtain Notifier(name (unnamed)="CODCr" ("名称（未命名）"), notification data type=FALSE) -> (notifier out=w363:refnum<notifier>, error out=w361:errorcluster)  [unwired: 2 in, 1 out]
            n204 = call "CODCrMB_api.vi"("STEP"=enum16{"open", "read", "write", "close"}."write", "values"=u16[] [12], "starting address"=u16 4608) -> ()  [unwired: 6 in, 3 out]
            n205 = Send Notification(notification=TRUE ("通知"), notifier=w363, error in (no error)=w361) -> (notifier out=w360:refnum<notifier>, error out=w359:errorcluster)
            n206 = Release Notifier(notifier=w360, error in (no error)=w359) -> ()  [unwired: 1 in, 3 out]
          }
        }
      }
      event "保存KB值": Value Change {
        n207 = event-data() -> ()  [unwired: 1 in, 6 out]
        n208 = local read "曲线斜率B"() -> (w373:sgl)
        n209 = local read "曲线斜率K"() -> (w374:sgl)
        n210 = Build Array(w374, w373) -> (w372:sgl[])
        n211 = call "FloatToHex.vi"("浮点数"=w372) -> ("DCBA整形输出"=w369:u16[])  [unwired: 10 in]
        n212 = call "CODCrMB_api.vi"("STEP"=enum16{"open", "read", "write", "close"}."write", "values"=w369, "starting address"=u16 4263) -> ()  [unwired: 6 in, 3 out]
      }
      event "定时启动": Value Change {
        n213 = event-data() -> ()  [unwired: 1 in, 6 out]
        n214 = flat-sequence {
          frame #0 {
            n215 = global read "CODcr全局变量.vi" "定时控制"() -> (w376:T7)
            n216 = call "周期设置.vi"("定时控制参数输入"=w376) -> ("定时控制参数输出"=w375:T7)  [unwired: 10 in]
            n217 = global write "CODcr全局变量.vi" "定时控制"(w375) -> ()
          }
          frame #1 {
            n218 = call <vilib>:"Application Directory.vi"() -> ("Application Directory"=w390:path)
            n219 = Build Path(base path=w390, name or relative path="data\\sys.ini" ("名称或相对路径")) -> (appended path=w388:path)
            n220 = call <vilib>:"Open Config Data.vi"("configuration file path"=w388) -> ("error out"=w384:errorcluster, "refnum"=w387:T10)  [unwired: 8 in, 1 out]
            n221 = vi-ref "CODCr库.lvlib:CODcr全局变量.vi"() -> (w386:refnum<vi>)
            n222 = call <userlib>:"Write Panel to INI__ogtk.vi"("error in (no error)"=w384, "VI ref"=w386, "refnum"=w387) -> ("error out"=w383:errorcluster, "refnum out"=w385:T10)  [unwired: 7 in]
            n223 = call <vilib>:"Close Config Data.vi"("error in (no error)"=w383, "refnum"=w385) -> ("error out"=w378:errorcluster, "file path"=w377:path)  [unwired: 8 in]
            n224 = Open/Create/Replace File(file path (use dialog)=w377, error in=w378) -> (refnum out=w381:refnum<file>, error out=w382:errorcluster)  [unwired: 4 in, 1 out]
            n225 = Flush File(refnum=w381, error in=w382) -> (refnum out=w380:refnum<file>, error out=w379:errorcluster)
            n226 = Close File(refnum=w380, error in=w379) -> ()  [unwired: 2 out]
          }
        }
      }
      event "仪器参数": Value Change {
        n227 = event-data() -> ()  [unwired: 1 in, 6 out]
        n228 = global read "CODcr全局变量.vi" "CODCr仪器参数"() -> (w392:T18)
        n229 = call "仪器参数设置.vi"("仪器参数设置"=w392) -> ("仪器参数设置输出"=w391:T19)  [unwired: 10 in]
        n230 = Unbundle By Name(w391) -> ("确定"=w393:bool)
        n231 = case shown="真" w393 {
          tunnel: w392 -> [_ w395]
          tunnel: w391 -> [_ w394]
          frame False {
          }
          frame True {
            n232 = flat-sequence {
              tunnel: w395 -> [w412]
              tunnel: w394 -> [w411]
              frame #0 {
                n233 = Unbundle By Name(w411) -> ("测量量程"=w410:dbl, "测量精度"=w409:dbl, "测量间隔"=w408:dbl, "消解温度"=w407:dbl, "消解时长"=w406:dbl, "空白校准时间"=w405:timestamp, "曲线截距"=w404:dbl, "曲线斜率"=w403:dbl, "测量检出限"=w402:dbl, "测量信号值"=w401:dbl, "线性相关系数"=w400:dbl, "二次多项式系数"=w399:dbl, "标样校准时间"=w398:timestamp, "单位"=w397:u16)
                n234 = Bundle By Name(cluster=w412, "测量量程"=w410, "测量精度"=w409, "测量间隔"=w408, "消解温度"=w407, "消解时长"=w406, "空白校准时间"=w405, "曲线截距"=w404, "曲线斜率"=w403, "测量检出限"=w402, "测量信号值"=w401, "线性相关系数"=w400, "二次多项式系数"=w399, "标样校准时间"=w398, "单位"=w397) -> (w396:T18)
                n235 = global write "CODcr全局变量.vi" "CODCr仪器参数"(w396) -> ()
              }
              frame #1 {
                n236 = call <vilib>:"Application Directory.vi"() -> ("Application Directory"=w426:path)
                n237 = Build Path(base path=w426, name or relative path="data\\sys.ini" ("名称或相对路径")) -> (appended path=w424:path)
                n238 = call <vilib>:"Open Config Data.vi"("configuration file path"=w424) -> ("error out"=w420:errorcluster, "refnum"=w423:T10)  [unwired: 8 in, 1 out]
                n239 = vi-ref "CODCr库.lvlib:CODcr全局变量.vi"() -> (w422:refnum<vi>)
                n240 = call <userlib>:"Write Panel to INI__ogtk.vi"("error in (no error)"=w420, "VI ref"=w422, "refnum"=w423) -> ("error out"=w419:errorcluster, "refnum out"=w421:T10)  [unwired: 7 in]
                n241 = call <vilib>:"Close Config Data.vi"("error in (no error)"=w419, "refnum"=w421) -> ("error out"=w414:errorcluster, "file path"=w413:path)  [unwired: 8 in]
                n242 = Open/Create/Replace File(file path (use dialog)=w413, error in=w414) -> (refnum out=w417:refnum<file>, error out=w418:errorcluster)  [unwired: 4 in, 1 out]
                n243 = Flush File(refnum=w417, error in=w418) -> (refnum out=w416:refnum<file>, error out=w415:errorcluster)
                n244 = Close File(refnum=w416, error in=w415) -> ()  [unwired: 2 out]
              }
            }
          }
        }
      }
      event "打开串口": Value Change {
        n245 = event-data() -> ()  [unwired: 1 in, 6 out]
        n246 = global read "CODcr全局变量.vi" "VISA Resource"() -> (w435:refnum<visa-resource-name>)
        n247 = global read "CODcr全局变量.vi" "PORT"() -> (w429:string)
        n248 = global read "CODcr全局变量.vi" "IP"() -> (w430:string)
        n249 = call "串口配置.vi"("PORT"=w429, "IP"=w430, "请选择串口:"=w435) -> ("PORT 2"=w431:string, "IP 2"=w432:string, "确认 2"=w434:bool, "VISA资源名称 2"=w433:refnum<visa-resource-name>)  [unwired: 5 in]
        n250 = case shown="真" w434 {
          tunnel: w433 -> [_ w438]
          tunnel: w428 -> [_ w440]
          tunnel: w427 -> [_ w439]
          tunnel: w432 -> [_ w437]
          tunnel: w431 -> [_ w436]
          frame False {
          }
          frame True {
            n251 = global write "CODcr全局变量.vi" "VISA Resource"(w438) -> ()
            n252 = global write "CODcr全局变量.vi" "PORT"(w436) -> ()
            n253 = global write "CODcr全局变量.vi" "IP"(w437) -> ()
            n254 = Bundle By Name(cluster=cluster{"命令":string} {"命令"=""} ("元素"), "命令"="启用模块" ("名称（未命名）")) -> (w441:cluster{"命令":string})
            n255 = Enqueue Element(queue=w440, element=w441, error in (no error)=w439) -> ()  [unwired: 1 in, 3 out]
          }
        }
      }
      event "释放串口": Value Change {
        n256 = event-data() -> ()  [unwired: 1 in, 6 out]
        n257 = Two Button Dialog(message="确认是否释放串口，释放串口将导致通信失败！" ("消息")) -> (T button?=w446:bool)  [unwired: 2 in]
        n258 = case shown="真" w446 {
          tunnel: w445 -> [_ w449]
          tunnel: w444 -> [_ w448]
          frame False {
          }
          frame True {
            n259 = Bundle By Name(cluster=cluster{"命令":string} {"命令"=""} ("元素"), "命令"="停用模块" ("名称（未命名）")) -> (w450:cluster{"命令":string})
            n260 = Enqueue Element(queue=w449, element=w450, error in (no error)=w448) -> ()  [unwired: 1 in, 3 out]
          }
        }
      }
      event "MB通信方式选择": Value Change {
        n261 = event-data() -> ()  [unwired: 1 in, 6 out]
        n262 = flat-sequence {
          frame #0 {
            n263 = global write "CODcr全局变量.vi" "MB通信方式选择"("MB通信方式选择") -> ()
          }
          frame #1 {
            n264 = call <vilib>:"Application Directory.vi"() -> ("Application Directory"=w467:path)
            n265 = Build Path(base path=w467, name or relative path="data\\sys.ini" ("名称或相对路径")) -> (appended path=w465:path)
            n266 = call <vilib>:"Open Config Data.vi"("configuration file path"=w465) -> ("error out"=w461:errorcluster, "refnum"=w464:T10)  [unwired: 8 in, 1 out]
            n267 = vi-ref "CODCr库.lvlib:CODcr全局变量.vi"() -> (w463:refnum<vi>)
            n268 = call <userlib>:"Write Panel to INI__ogtk.vi"("error in (no error)"=w461, "VI ref"=w463, "refnum"=w464) -> ("error out"=w460:errorcluster, "refnum out"=w462:T10)  [unwired: 7 in]
            n269 = call <vilib>:"Close Config Data.vi"("error in (no error)"=w460, "refnum"=w462) -> ("error out"=w455:errorcluster, "file path"=w454:path)  [unwired: 8 in]
            n270 = Open/Create/Replace File(file path (use dialog)=w454, error in=w455) -> (refnum out=w458:refnum<file>, error out=w459:errorcluster)  [unwired: 4 in, 1 out]
            n271 = Flush File(refnum=w458, error in=w459) -> (refnum out=w457:refnum<file>, error out=w456:errorcluster)
            n272 = Close File(refnum=w457, error in=w456) -> ()  [unwired: 2 out]
          }
        }
      }
      event "写入消解温度时长": Value Change {
        n273 = event-data() -> ()  [unwired: 1 in, 6 out]
        n274 = local read "消解时长"() -> (w472:u16)
        n275 = local read "消解温度"() -> (w473:u16)
        n276 = Build Array(w473, w472) -> (w471:u16[])
        n277 = call "WordToHex.vi"("WORD"=w471) -> ("数组"=w468:u16[])  [unwired: 10 in]
        n278 = call "CODCrMB_api.vi"("STEP"=enum16{"open", "read", "write", "close"}."write", "values"=w468, "starting address"=u16 4257) -> ()  [unwired: 6 in, 3 out]
      }
      event "校时": Value Change {
        n279 = event-data() -> ()  [unwired: 1 in, 6 out]
        n280 = Get Date/Time In Seconds() -> (seconds since 1Jan1904=w481:timestamp)
        n281 = Build Array(w481) -> (w478:timestamp[])
        n282 = call "DateToHex.vi"("DATE"=w478) -> ("数组"=w477:u16[])  [unwired: 10 in]
        n283 = Insert Into Array(array=u16[] [13] ("values"), index=1 ("索引"), new element=w477) -> (w474:u16[])
        n284 = call "CODCrMB_api.vi"("STEP"=enum16{"open", "read", "write", "close"}."write", "values"=w474, "starting address"=u16 4608) -> ()  [unwired: 6 in, 3 out]
      }
      event "设置": Value Change {
        n285 = event-data() -> ()  [unwired: 1 in, 6 out]
        n286 = property on="窗格" class="Pane"("Origin"=T9 {"Horizontal"=0, "Vertical"=728} ("原点")) -> ()  [unwired: 2 in, 2 out]
        n287 = Bundle By Name(cluster=cluster{"命令":string} {"命令"=""} ("元素"), "命令"="CODCr读取参数" ("名称（未命名）")) -> (w484:cluster{"命令":string})
        n288 = Enqueue Element(queue=w483, element=w484, error in (no error)=w482) -> ()  [unwired: 1 in, 3 out]
      }
      event "返回": Value Change {
        w488 = FALSE ("可见")
        n289 = event-data() -> ()  [unwired: 1 in, 6 out]
        n290 = property on="窗格" class="Pane"("Origin"=T9 {"Horizontal"=0, "Vertical"=0} ("原点")) -> ()  [unwired: 2 in, 2 out]
        n291 = property on="写入消解温度时长" class="Bool"("Visible"=w488) -> ()  [unwired: 2 in, 2 out]
        n292 = property on="释放串口" class="Bool"("Visible"=w488) -> ()  [unwired: 2 in, 2 out]
        n293 = property on="打开串口" class="Bool"("Visible"=w488) -> ()  [unwired: 2 in, 2 out]
        n294 = property on="MB通信方式选择" class="Enum (严格)"("Visible"=w488) -> ()  [unwired: 2 in, 2 out]
      }
      event "曲线斜率K", "曲线斜率B", "消解温度", "消解时长": Mouse Down {
        n295 = event-data() -> ("CtlRef"=w492:refnum<vi>)  [unwired: 1 in, 7 out]
        n296 = property class="DigNum"(reference=w492) -> (reference out=w493:refnum<vi>, "Value"=w491:variant)  [unwired: 1 in, 1 out]
        n297 = Variant To Data(Variant=w491) -> (data=w490:sgl)  [unwired: 2 in, 1 out]
        n298 = call "CODCR数字键盘.vi"("OldNumber"=w490) -> ("NewNumber"=w494:sgl)
        n299 = property class="DigNum"(reference=w493, "Value"=w494) -> ()  [unwired: 1 in, 2 out]
      }
      event "隐藏按钮": Value Change {
        w495 = TRUE ("可见")
        n300 = event-data() -> ()  [unwired: 1 in, 6 out]
        n301 = property on="写入消解温度时长" class="Bool"("Visible"=w495) -> ()  [unwired: 2 in, 2 out]
        n302 = property on="释放串口" class="Bool"("Visible"=w495) -> ()  [unwired: 2 in, 2 out]
        n303 = property on="打开串口" class="Bool"("Visible"=w495) -> ()  [unwired: 2 in, 2 out]
        n304 = property on="MB通信方式选择" class="Enum (严格)"("Visible"=w495) -> ()  [unwired: 2 in, 2 out]
      }
    }
  }
  n305 = while {
    tunnel: w2 -> [w497]
    tunnel: w1 -> [w496]
    i -> [w505]
    stop <- FALSE stop-if-true
    n306 = First Call?() -> (First Call?: T/F=w500:bool)
    n307 = case shown="真" w500 {
      tunnel: w497 -> [w509 w514]
      tunnel: w496 -> [w508 w513]
      tunnel: [w509 w512] -> w499
      tunnel: [w508 w511] -> w498
      frame False {
      }
      frame True {
        n308 = Bundle By Name(cluster=cluster{"命令":string} {"命令"=""} ("元素"), "命令"="CODMn读取参数" ("名称（未命名）")) -> (w517:cluster{"命令":string})
        n309 = Enqueue Element(queue=w514, element=w517, timeout in ms (-1)=1000 ("超时毫秒(-1)"), error in (no error)=w513) -> (queue out=w512:refnum<queue>, error out=w511:errorcluster)  [unwired: 1 out]
      }
    }
    n310 = Get Queue Status(queue=w499, error in (no error)=w498) -> (queue out=w503:refnum<queue>, error out=w502:errorcluster, # elements in queue=w504:i32)  [unwired: 1 in, 5 out]
    n311 = Equal To 0?(x=w504) -> (x = 0?=w501:bool)
    n312 = case shown="真" w501 {
      tunnel: w503 -> [_ w519]
      tunnel: w502 -> [_ w518]
      frame False {
      }
      frame True {
        n313 = Bundle By Name(cluster=cluster{"命令":string} {"命令"=""} ("元素"), "命令"="CODCr读取" ("名称（未命名）")) -> (w521:cluster{"命令":string})
        n314 = Enqueue Element(queue=w519, element=w521, timeout in ms (-1)=1000 ("超时毫秒(-1)"), error in (no error)=w518) -> ()  [unwired: 3 out]
      }
    }
    n315 = Wait (ms)(milliseconds to wait=u32 1000 ("等待时间（毫秒）")) -> ()  [unwired: 1 out]
    "主循环次数" <- w505
  }
